vi "GetRotatedACPadError.vi"() -> ()   [LabVIEW 2018]
uses:
  <vilib>/userdefined/High Color/IMAQdx.ctl
  <vilib>/Utility/file.llb/Read Delimited Spreadsheet (DBL).vi
  <vilib>/Utility/file.llb/Read Delimited Spreadsheet (I64).vi
  <vilib>/Utility/file.llb/Write Delimited Spreadsheet (DBL).vi
  <vilib>/vision/driver/NI_Vision_Acquisition_Software.lvlib
  <vilib>/vision/NI_Vision_Development_Module.lvlib
panel:
  in  "Sensor":string(combo)="R0Hamamatsu"
  out "Pattern Matched Image":T1(plugin-control)
  in  "Begin":bool
  out "Image Out":T1(plugin-control)
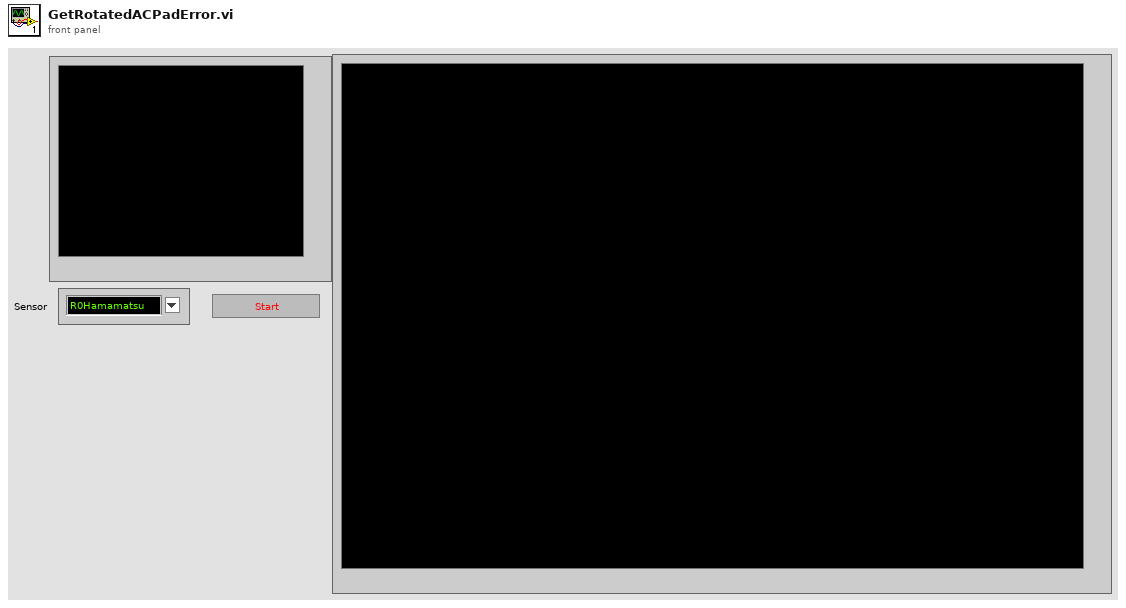
[diagram p1: front panel]
types:
  T1 = typedef "IMAQ Image.ctl" = refnum<image>
  T2 = typedef "Image Type" = u32
  T3 = typedef "IMAQdx.ctl" = refnum<k21>
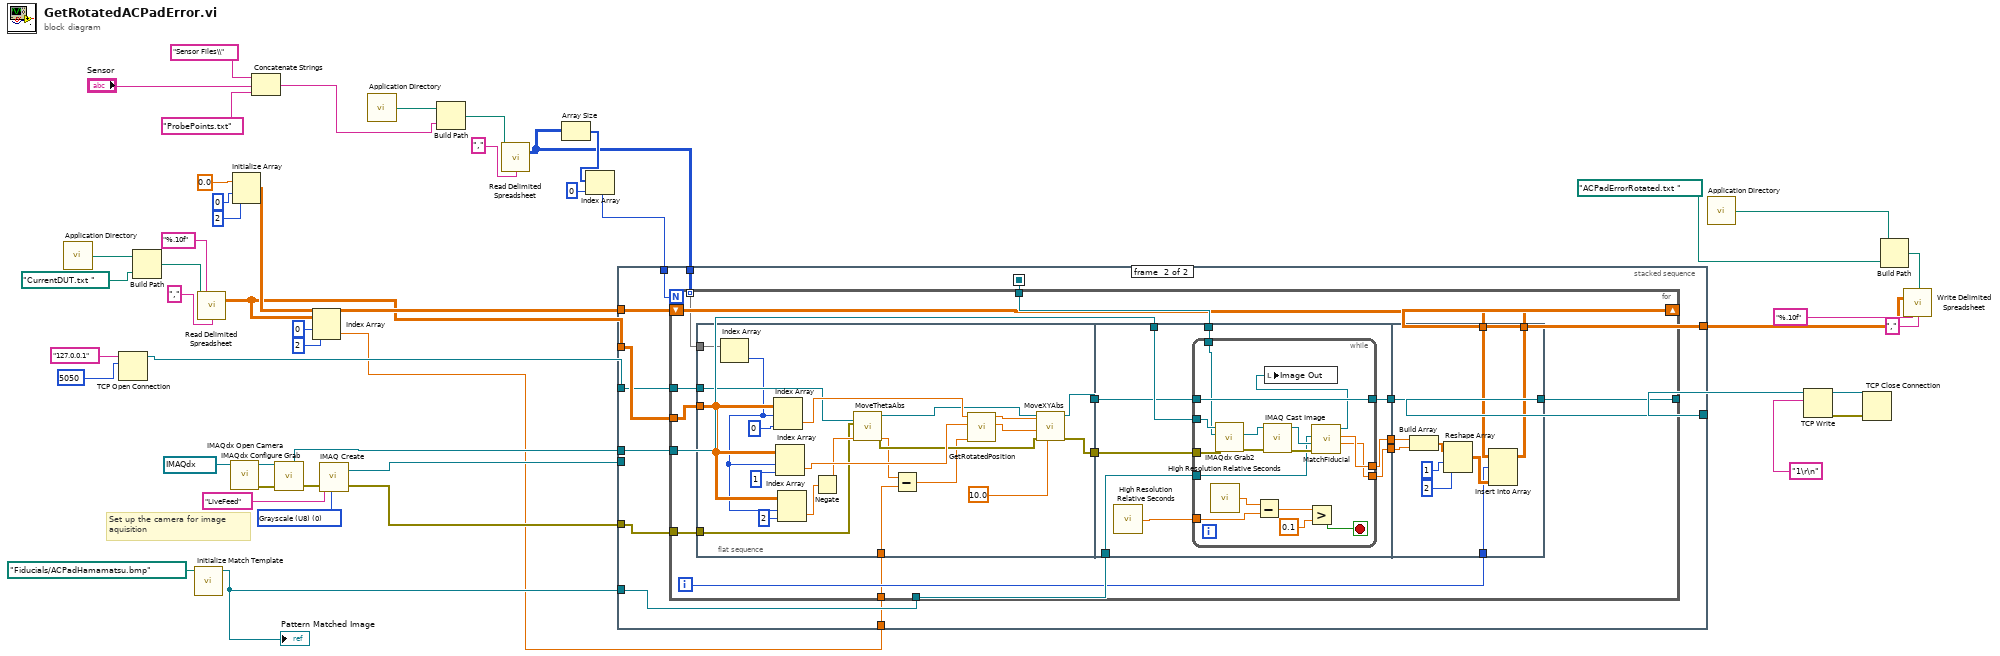
[diagram p0: block diagram]
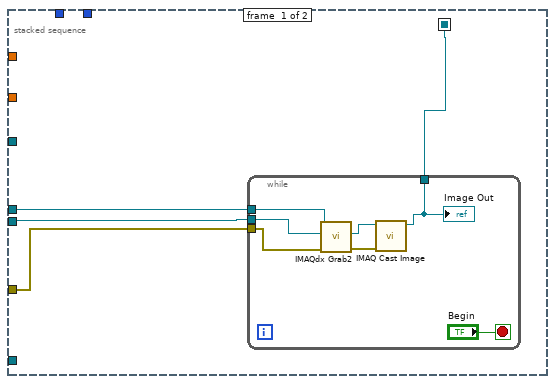
[diagram p2: hidden frame]
diagram:
  w38 = T2 0 items=["Grayscale (U8)", "Grayscale (I16)", "Grayscale (SGL)", "Complex (CSG)", "RGB (U32)", "HSL (U32)", "RGB (U64)", "Grayscale (U16)"] ("Image Type")
  # "Set up the camera for image \naquisition"
  n1 = call <vilib>:"Application Directory.vi"() -> ("Application Directory"=w45:path)
  n2 = TCP Open Connection(address="127.0.0.1", remote port or service name=u16 5050) -> (connection ID=w6:refnum<k5>)  [unwired: 3 in, 1 out]
  n3 = Build Path(base path=w45, name or relative path=path "CurrentDUT.txt " ("file path (dialog if empty)")) -> (appended path=w46:path)
  n4 = call "Initialize Match Template.vi"("base path"=path "Fiducials/ACPadHamamatsu.bmp") -> ("Pattern Matched Image"=w17:T1)  [unwired: 10 in]
  "Pattern Matched Image" <- w17
  n5 = call-poly <vilib>:"Read Delimited Spreadsheet.vi"("file path (dialog if empty)"=w46, "format (%.3f)"="%.10f", "delimiter (\\t)"="," ("delimiter (\\t)")) -> ("all rows"=w9:dbl[][])  [unwired: 7 in, 5 out]
  n6 = call <vilib>:"IMAQdx Open Camera.vi"("Session In"=T3 "cam0") -> ("error out"=w41:errorcluster, "Session Out"=w42:T3)  [unwired: 9 in]
  n7 = Initialize Array(0.0 ("element"), 0 ("dimension size"), 2 ("dimension size")) -> (w25:dbl[][])
  n8 = Concatenate Strings("Sensor Files\\" ("string"), "Sensor", "ProbePoints.txt" ("string")) -> (w2:string)
  n9 = call <vilib>:"IMAQdx Configure Grab.vi"("error in"=w41, "Session In"=w42) -> ("error out"=w39:errorcluster, "Session Out"=w37:T3)  [unwired: 8 in]
  n10 = Index Array(array=w9, index (row)=0, index (col)=2 ("disabled index (col)")) -> (element=w5:dbl)
  n11 = call "IMAQ Create"("Image Name"="LiveFeed", "Image Type"=w38, "error in (no error)"=w39) -> ("New Image"=w36:T1, "error out"=w35:errorcluster)  [unwired: 2 in]
  n12 = call <vilib>:"Application Directory.vi"() -> ("Application Directory"=w14:path)
  n13 = Build Path(base path=w14, name or relative path=w2) -> (appended path=w15:path)
  n14 = call-poly <vilib>:"Read Delimited Spreadsheet.vi"("file path (dialog if empty)"=w15, "delimiter (\\t)"="," ("delimiter (\\t)")) -> ("all rows"=w10:i64[][])  [unwired: 8 in, 5 out]
  n15 = Array Size(array=w10) -> (size(s)=w13:i32[])
  n16 = Index Array(array=w13, index=0) -> (element=w11:i32)
  n17 = stacked-sequence {
    seq-local: [w49 _] -> [_ w70]
    tunnel: w17 -> [_ w71]
    tunnel: w37 -> [w52 w69]
    tunnel: w36 -> [w51 _]
    tunnel: w35 -> [w50 w61]
    tunnel: w9 -> [_ w66]
    tunnel: [_ w68] -> w26
    tunnel: w25 -> [_ w67]
    tunnel: w6 -> [_ w65]
    tunnel: [_ w64] -> w18
    tunnel: w11 -> [_ w63]
    tunnel: w10 -> [_ w62]
    tunnel: w5 -> [_ w60]
    frame #0 {
      n18 = while {
        tunnel: w52 -> [w58]
        tunnel: w50 -> [w57]
        tunnel: w51 -> [w56]
        tunnel: [w53] -> w49
        stop <- "Begin" stop-if-true
        n19 = call <vilib>:"IMAQdx Grab2.vi"("error in"=w57, "Image In"=w56, "Session In"=w58) -> ("error out"=w54:errorcluster, "Image Out"=w55:T1)  [unwired: 5 in, 2 out]
        n20 = call "IMAQ Cast Image"("error in (no error)"=w54, "Image Src"=w55) -> ("Image Dst Out"=w53:T1)  [unwired: 8 in, 1 out]
        "Image Out" <- w53
      }
    }
    frame #1 {
      n21 = for {
        N: w63 -> [_]
        tunnel: w71 -> [w88]
        tunnel: w70 -> [w87]
        tunnel: w69 -> [w86]
        shift-right: [w83] -> w68
        shift-left: w67 -> [w82]
        tunnel: w66 -> [w81]
        tunnel: w65 -> [w79]
        tunnel: [w75] -> w64
        tunnel: w62 -> [w74] mode=indexing
        tunnel: w61 -> [w73]
        tunnel: w60 -> [w72]
        i -> [w80]
        n22 = flat-sequence {
          tunnel: w81 -> [w105]
          tunnel: w79 -> [w94]
          tunnel: [w108] -> w78
          tunnel: [w107] -> w77
          tunnel: w74 -> [w106]
          tunnel: w73 -> [w95]
          tunnel: w72 -> [w92]
          tunnel: w88 -> [w118]
          tunnel: w87 -> [w117]
          tunnel: w86 -> [w116]
          tunnel: [w114] -> w85
          tunnel: [w115] -> w84
          tunnel: w78 -> [w113]
          tunnel: w77 -> [w112]
          tunnel: [w111] -> w76
          tunnel: [w144] -> w83
          tunnel: w85 -> [w143]
          tunnel: w84 -> [w142]
          tunnel: w80 -> [w141]
          tunnel: w82 -> [w138]
          tunnel: [w137] -> w75
          tunnel: w76 -> [w137]
          frame #0 {
            n23 = Index Array(array=w106) -> (element=w89:i64)  [unwired: 1 in]
            n24 = Index Array(array=w105, index (row)=w89, index (col)=0 ("index")) -> (element=w102:dbl)
            n25 = Index Array(array=w105, index (row)=w89, index (col)=1 ("index")) -> (element=w103:dbl)
            n26 = Index Array(array=w105, index (row)=w89, index (col)=2 ("disabled index (col)")) -> (element=w93:dbl)
            n27 = Negate(x=w93) -> (-x=w97:dbl)
            n28 = call "MoveThetaAbs.vi"("Theta"=w97, "error out 2"=w95, "connection ID"=w94) -> ("ThetaOut (rad)"=w91:dbl, "error out"=w98:errorcluster, "connection ID 2"=w99:refnum<k5>)  [unwired: 6 in]
            n29 = Subtract(x=w91, y=w92) -> (x-y=w90:dbl)
            n30 = call "GetRotatedPosition.vi"("theta"=w90, "Y"=w103, "X"=w102) -> ("Y'"=w100:dbl, "X'"=w101:dbl)  [unwired: 7 in]
            n31 = call "MoveXYAbs.vi"("%Speed"=10.0, "error in (no error) 2"=w98, "Y"=w100, "X"=w101, "connection ID 2"=w99) -> ("error out"=w108:errorcluster, "connection ID"=w107:refnum<k5>)  [unwired: 5 in]
          }
          frame #1 {
            n32 = call <vilib>:"High Resolution Relative Seconds.vi"() -> ("relative seconds"=w119:dbl)
            n33 = while {
              tunnel: w119 -> [w133]
              tunnel: w118 -> [w122]
              tunnel: w113 -> [w127]
              tunnel: w117 -> [w126]
              tunnel: w116 -> [w136]
              tunnel: [w130] -> w114
              tunnel: [w129] -> w115
              tunnel: w112 -> [w128]
              tunnel: [w128] -> w111
              stop <- w135 stop-if-true
              n34 = call <vilib>:"High Resolution Relative Seconds.vi"() -> ("relative seconds"=w134:dbl)
              n35 = call <vilib>:"IMAQdx Grab2.vi"("error in"=w127, "Image In"=w126, "Session In"=w136) -> ("error out"=w125:errorcluster, "Image Out"=w120:T1)  [unwired: 5 in, 2 out]
              n36 = Subtract(x=w134, y=w133) -> (x-y=w132:dbl)
              n37 = call "IMAQ Cast Image"("error in (no error)"=w125, "Image Src"=w120) -> ("error out"=w124:errorcluster, "Image Dst Out"=w123:T1)  [unwired: 8 in]
              n38 = Greater?(x=w132, y=0.1) -> (0:w135:bool)
              n39 = call "MatchFiducial.vi"("error in"=w124, "Image In"=w123, "Template Image"=w122) -> ("Y (um)"=w129:dbl, "X (um)"=w130:dbl, "Image Out"=w121:T1)  [unwired: 3 in, 3 out]
              n40 = local write "Image Out"(w121) -> ()
            }
          }
          frame #2 {
            n41 = Build Array(w143, w142) -> (w146:dbl[])
            n42 = Reshape Array(w146, 1 ("dimension size"), 2 ("dimension size")) -> (w145:dbl[][])
            n43 = Insert Into Array(array=w138, index (row)=w141, new element=w145) -> (w144:dbl[][])  [unwired: 1 in]
          }
        }
      }
    }
  }
  n44 = call <vilib>:"Application Directory.vi"() -> ("Application Directory"=w30:path)
  n45 = TCP Write(connection ID=w18, data in="1\r\n") -> (connection ID out=w20:refnum<k5>, error out=w21:errorcluster)  [unwired: 2 in, 1 out]
  n46 = TCP Close Connection(connection ID=w20, error in (no error)=w21) -> ()  [unwired: 1 in, 2 out]
  n47 = Build Path(base path=w30, name or relative path=path "ACPadErrorRotated.txt " ("file path (dialog if empty)")) -> (appended path=w29:path)
  n48 = call-poly <vilib>:"Write Delimited Spreadsheet.vi"("file path (dialog if empty)"=w29, "format (%.3f)"="%.10f", "2D data"=w26, "delimiter (\\t)"="," ("delimiter (\\t)")) -> ()  [unwired: 10 in, 2 out]
